vi "Measure I-V of Diodes.vi"(0 "AO Task In":refnum<k21>, 1 "AI Task In":refnum<k21>, 2 "V_App Array":dbl[](array[numeric]), 3 "I/O Array In":dbl[][](array[numeric]), 4 "# pts":dbl, 5 "index":i32, 6 "Delay":dbl, 7 "R_Ref":dbl) -> (14 "AO Task Out":refnum<k21>, 15 "AI Task Out":refnum<k21>, 16 "I/O Array Out":dbl[][](array[numeric]), 17 "X Input":dbl, 18 "Y Input":dbl, 19 "error out":errorcluster)   [LabVIEW 2020]
doc: "Measure I-V of Diodes.vi writes an inputted voltage to the NI myDAQ channel AO0, waits for an inputted delay time, reads the voltage across a reference resistor through AI0, reads the voltage across a diode through AI1, then as output appends these measurements to a double numeric array of outputted voltages, calculated currents, and measured diode voltages."
uses:
  <vilib>/DAQmx/write.llb/DAQmx Write (Analog DBL 1Chan 1Samp).vi
  <vilib>/DAQmx/read.llb/DAQmx Read (Analog 1D DBL NChan 1Samp).vi
  <vilib>/DAQmx/miscellaneous.llb/DAQmx Fill In Error Info.vi
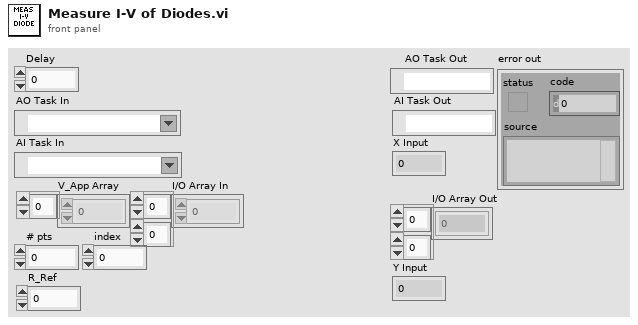
[diagram p1: front panel]
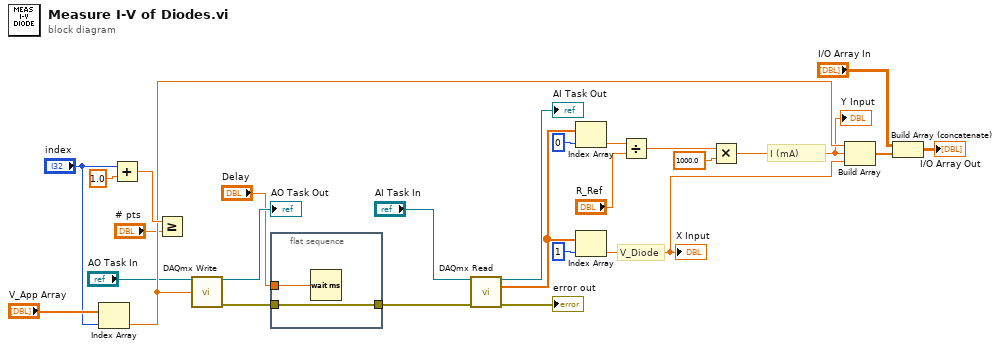
[diagram p0: block diagram]
diagram:
  # "I (mA)"
  # "V_Diode"
  n1 = Index Array(array="V_App Array", index="index") -> (element=w16:dbl)
  n2 = Add(x="index", y=1.0) -> (x+y=w20:dbl)
  n3 = Greater Or Equal?(x=w20, y="# pts") -> ()  [unwired: 1 out]
  n4 = call-poly <vilib>:"DAQmx Write.vi"("task/channels in"="AO Task In", "data"=w16) -> ("task out"=→"AO Task Out":refnum<k21>, "error out"=w25:errorcluster)  [unwired: 11 in, 1 out]
  n5 = flat-sequence {
    tunnel: w25 -> [w28]
    tunnel: [w28] -> w24
    tunnel: "Delay" -> [w27]
    frame #0 {
      n6 = Wait (ms)(milliseconds to wait=w27) -> ()  [unwired: 1 out]
    }
  }
  n7 = call-poly <vilib>:"DAQmx Read.vi"("task/channels in"="AI Task In", "error in"=w24) -> ("task out"=→"AI Task Out":refnum<k21>, "data"=w18:dbl[], "error out"=→"error out":errorcluster)  [unwired: 11 in]
  n8 = Index Array(array=w18, index=0) -> (element=w13:dbl)
  n9 = Index Array(array=w18, index=1) -> (element=w10:dbl)
  "X Input" <- w10
  n10 = Divide(x=w13, y="R_Ref") -> (x/y=w11:dbl)
  n11 = Multiply(x=w11, y=1000.0) -> (x*y=w9:dbl)
  "Y Input" <- w9
  n12 = Build Array(w16, w9, w10) -> (w15:dbl[])
  n13 = Build Array (concatenate)("I/O Array In", w15) -> (→"I/O Array Out":dbl[][])
